vi "Receive Observer Boradcasting.vi"(8 "error in (no error)":errorcluster, 10 "Boradcasting Data":variant, 11 "Subscriber in":refnum<class "Subscriber.lvclass">) -> (0 "error out":errorcluster, 3 "Subscriber out":refnum<class "Subscriber.lvclass">)   [LabVIEW 2019, in "Subscriber.lvclass"]
uses:
  Subscriber.lvclass
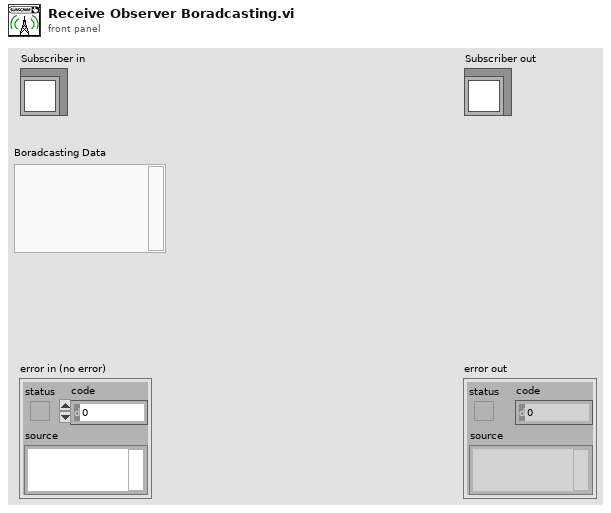
[diagram p1: front panel]
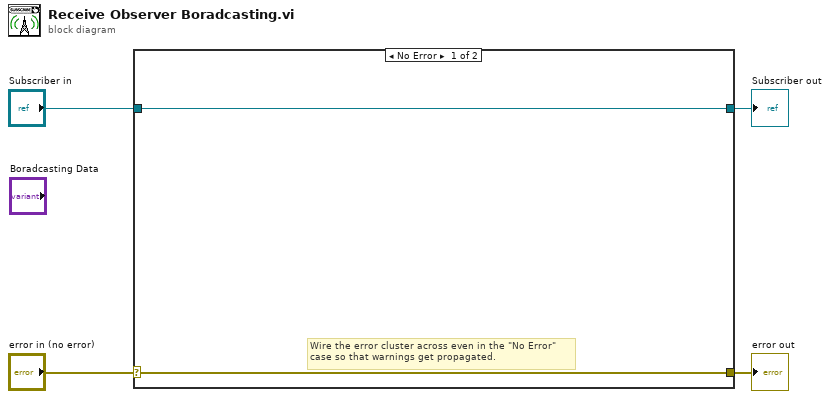
[diagram p0: block diagram]
diagram:
  n1 = case shown="No Error" "error in (no error)" {
    selector: "error in (no error)" -> [w5 w8]
    tunnel: [w5 w8] -> w3
    tunnel: [w6 w7] -> w1
    tunnel: "Subscriber in" -> [w6 w7]
    frame No Error {
      # "Wire the error cluster across even in the \"No Error\"\ncase so that warnings get propagated."
    }
    frame Error {
    }
  }
  "error out" <- w3
  "Subscriber out" <- w1
